vi "x_axis_pid_v5.vi"(10 "PID Gains":T1={"Proportional Gain (Kc)"=0.8, "Integral Gain"=25.0, "Derivative Gain"=0.004}, 11 "Gx, Gy, wz":dbl[](array[numeric])) -> (0 "Motor 4":dbl, 1 "Motor 3":dbl, 2 "Motor 2":dbl, 3 "Motor 1":dbl, 4 "error out":errorcluster)   [LabVIEW 2019]
uses:
  <vilib>/myRIO/Common/Instrument Driver Framework/myRIO v1.0/UART/vis/myRIO v1.0 Close UART.vi
  <vilib>/addons/control/pid/pid.llb/PID (DBL).vi
  <vilib>/myRIO/Common/Instrument Driver Framework/Utilities/vis/FPGA Ref Manager.vi
  <vilib>/myRIO/Common/Instrument Driver Framework/myRIO v1.0/myRIO v1.0 Reset FPGA.vi
  <vilib>/myRIO/Common/Instrument Driver Framework/myRIO v1.0/IRQ/vis/myRIO v1.0 IRQ Info FGV.vi
  <vilib>/myRIO/Common/Instrument Driver Framework/myRIO v1.0/IRQ/vis/myRIO v1.0 Timer IRQ Info FGV.vi
  <vilib>/myRIO/Common/Instrument Driver Framework/myRIO v1.0/IRQ/vis/myRIO v1.0 ISR Agent.vi
  <vilib>/myRIO/Instrument Drivers/Utilities/vis/Reset Index.vi
  <vilib>/myRIO/Common/Instrument Driver Framework/myRIO v1.0/Resource Manager/vis/myRIO v1.0 Block Write Resource Manager.vi
  <vilib>/addons/control/pid/NI_PID_pid.lvlib
  <vilib>/myRIO/Instrument Drivers/Utilities/Utilities.lvlib
panel:
  out "PID Out":dbl=1.8829840965238862 format="%0#4.1g"
  in  "Reinitialize":bool
  in  "stop":bool
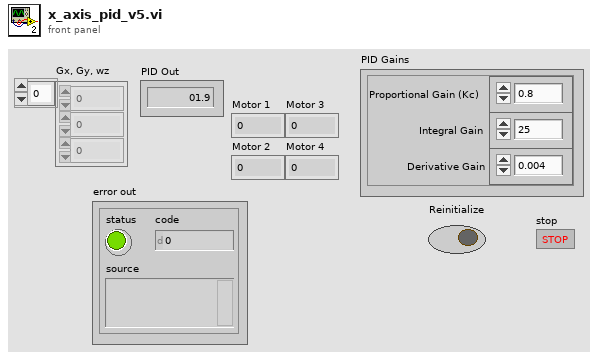
[diagram p1: front panel]
types:
  T1 = cluster{"Proportional Gain (Kc)":dbl, "Integral Gain":dbl, "Derivative Gain":dbl}
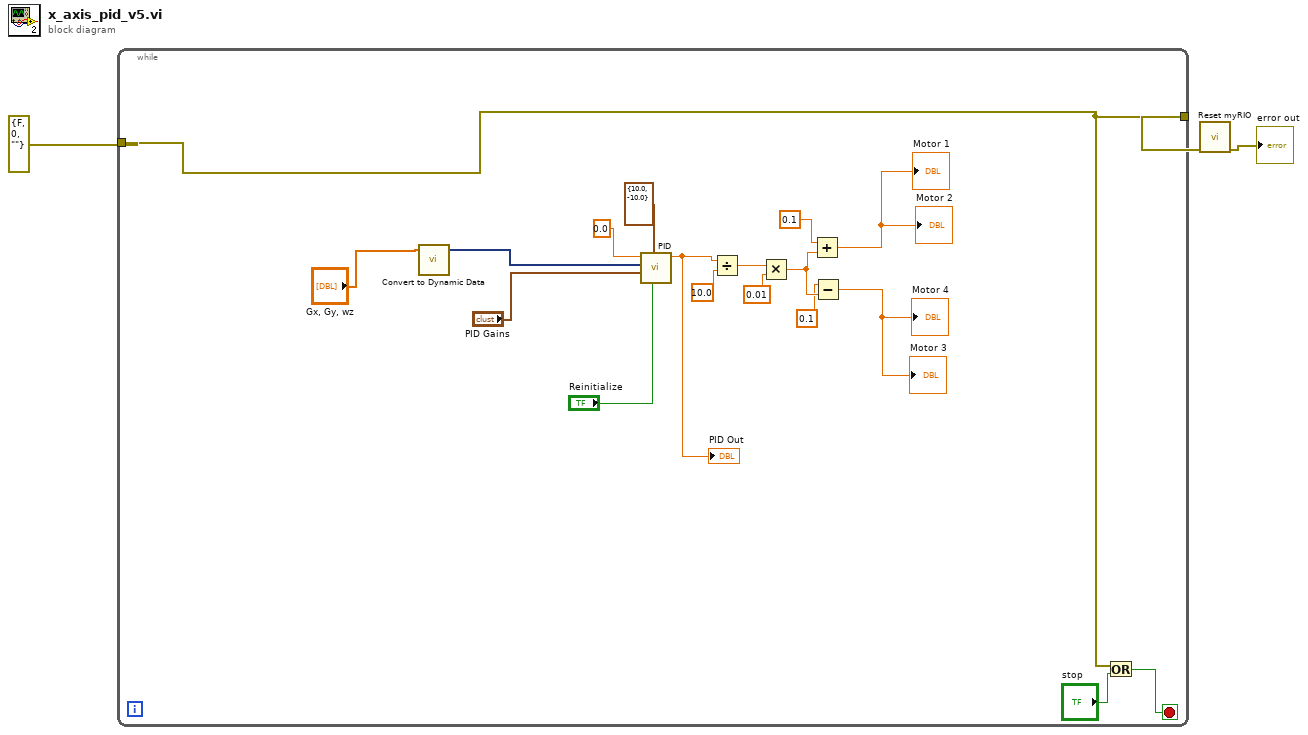
[diagram p0: block diagram]
diagram:
  n1 = while {
    tunnel: [w8] -> w3
    tunnel: errorcluster {"status"=FALSE, "code"=0, "source"=""} ("error in (no error)") -> [w8]
    stop <- w9 stop-if-true
    n2 = call "Convert to Dynamic Data"("Array"="Gx, Gy, wz") -> ("Dynamic Data Type"=w6:dynamicdata)  [unwired: 3 in]
    n3 = call-poly <vilib>:"PID.vi"("reinitialize? (F)"="Reinitialize", "output range"=cluster{"output high":dbl, "output low":dbl} {"output high"=10.0, "output low"=-10.0}, "PID gains"="PID Gains", "process variable"=w6, "setpoint"=0.0 ("Angle (rads)")) -> ("output"=w13:dbl)  [unwired: 5 in, 1 out]
    "PID Out" <- w13
    n4 = Divide(x=w13, y=10.0) -> (x/y=w20:dbl)
    n5 = Multiply(x=w20, y=0.01) -> (x*y=w19:dbl)
    n6 = Add(x=0.1, y=w19) -> (x+y=→"Motor 1" →"Motor 2":dbl)
    n7 = Subtract(x=0.1, y=w19) -> (x-y=→"Motor 3" →"Motor 4":dbl)
    n8 = Or(x=w8, y="stop") -> (x .or. y?=w9:bool)
  }
  n9 = call <vilib>:"Reset myRIO.vi"("error in (no error)"=w3) -> ("error out"=→"error out":errorcluster)  [unwired: 10 in]
